vi "Parallel Executing Test Code.vi"(9 "Test Complete Event":refnum<user-event>, 10 "Positions":u32[](array[numeric]), 11 "Example Parallel Test in":refnum<class "Example Parallel Test.lvclass">) -> ()   [LabVIEW 2015, in "Example Parallel Test.lvclass"]
uses:
  Example Parallel Test.lvclass
  Parallel Test/typedefs/Parallel Return -- Cluster.ctl
  Parallel Test/Parallel Test.lvclass
panel:
  in  "Fail":bool
  in  "Pass":bool
  out "String":string
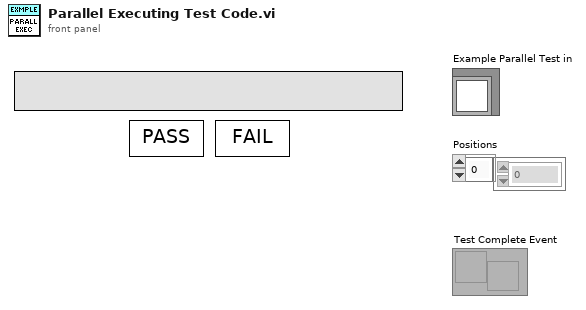
[diagram p1: front panel]
types:
  T1 = typedef "Parallel Test.lvclass/Parallel Return -- Cluster.ctl" = cluster{"Status":bool[], "Code":i32, "Source":string, "Position":u32[]}
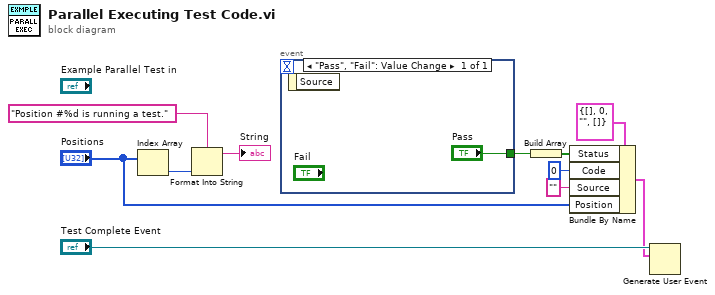
[diagram p0: block diagram]
diagram:
  n1 = Index Array(array="Positions") -> (element=w9:u32)  [unwired: 1 in]
  n2 = Format Into String(format string="Position #%d is running a test.", w9) -> (resulting string=→"String":string)  [unwired: 2 in, 1 out]
  n3 = event shown="[0] \"Pass\", \"Fail\": Value Change" {
    selector: _ -> [_]
    dyn-events: _ -> [_]
    timeout: _ -> [_]
    tunnel: ["Pass"] -> w4
    event "Pass", "Fail": Value Change {
      n4 = event-data() -> ()  [unwired: 1 in, 1 out]
    }
  }
  n5 = Build Array(w4) -> (w1:bool[])
  n6 = Bundle By Name(cluster=T1 {"Status"=[], "Code"=0, "Source"="", "Position"=[]} ("error IO"), "Status"=w1, "Code"=0 ("code"), "Source"="" ("source"), "Position"="Positions") -> (w6:T1)
  n7 = Generate User Event(user event="Test Complete Event", event data cluster=w6) -> ()  [unwired: 2 in, 2 out]
